vi "Set JSON Config.vi"(8 "error in (no error)":errorcluster, 10 "JSON Config":string, 11 "object in":refnum<class "Configuration Base.lvclass">) -> (0 "error out":errorcluster, 3 "object out":refnum<class "Configuration Base.lvclass">)   [LabVIEW 2023, in "Configuration Base.lvlib" / "Configuration Base.lvclass"]
uses:
  Configuration Base.lvclass
  Configuration Base.lvclass/Configuration Base.ctl
  D:/git/HAL/Configuration Base/Configuration Base.lvclass
  D:/git/HAL/HAL GOOP4/Interfaces/IConfigure/IConfigure.lvclass
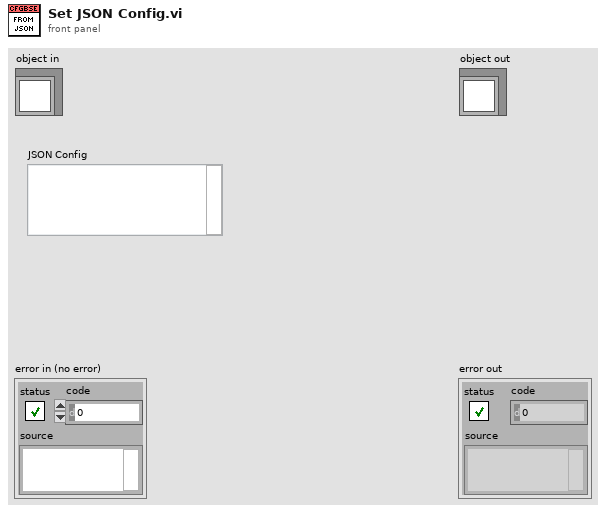
[diagram p1: front panel]
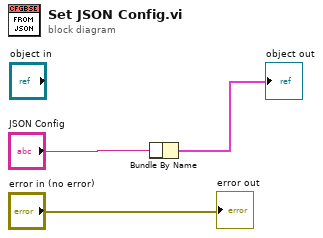
[diagram p0: block diagram]
diagram:
  n1 = Bundle By Name(cluster="JSON Config") -> (→"object out":cluster{})  [unwired: 1 in]
  "error out" <- "error in (no error)"
